vi "CRYStimulus Freq Max Limit.vi"(8 "Resolution":u16(ring) items=["R10 (1/3 Oct.)", "R20 (1/6 Oct.)", "R40 (1/12 Oct.)", "R80 (1/24 Oct.)", "User Defined, Log", "User Defined, Linear"], 9 "Decrement Flag":bool, 10 "Max Freq":dbl, 11 "Input Val":dbl) -> (2 "Decrement Val":dbl, 3 "Output Val":dbl)   [LabVIEW 2013]
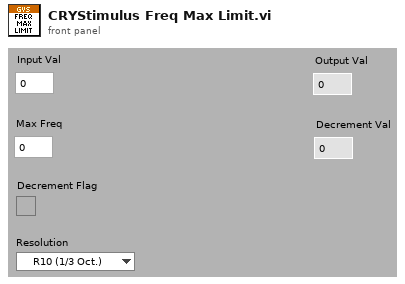
[diagram p1: front panel]
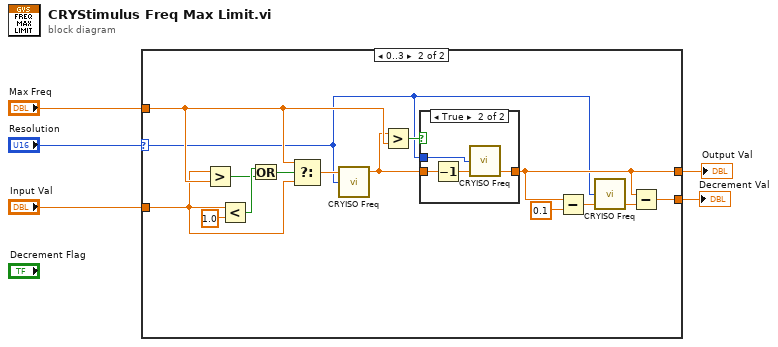
[diagram p0: block diagram]
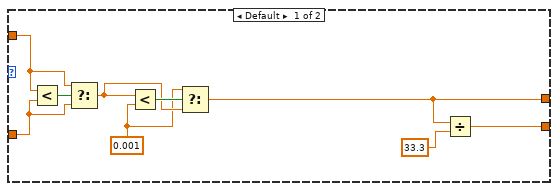
[diagram p2: hidden frame]
diagram:
  n1 = case shown="0..3" "Resolution" {
    selector: "Resolution" -> [_ w15]
    tunnel: [w6 w26] -> w5
    tunnel: [w8 w25] -> w4
    tunnel: "Max Freq" -> [w12 w23]
    tunnel: "Input Val" -> [w11 w22]
    frame Default {
      w9 = 0.001 ("y")
      n2 = Less?(x=w12, y=w11) -> (x < y?=w13:bool)
      n3 = Select(t=w12, s=w13, f=w11) -> (s? t:f=w10:dbl)
      n4 = Less?(x=w10, y=w9) -> (x < y?=w14:bool)
      n5 = Select(t=w9, s=w14, f=w10) -> (s? t:f=w8:dbl)
      n6 = Divide(x=w8, y=33.3) -> (x/y=w6:dbl)
    }
    frame 0..3 {
      n7 = Greater?(x=w22, y=w23) -> (0:w27:bool)
      n8 = Less?(x=w22, y=1.0) -> (x < y?=w28:bool)
      n9 = Or(x=w28, y=w27) -> (x .or. y?=w24:bool)
      n10 = Select(t=w23, s=w24, f=w22) -> (s? t:f=w21:dbl)
      n11 = call "CRYISO Freq.vi"("ISO series"=w15, "Higher Freq"=w21) -> ("Higher ISO Freq"=w19:dbl)  [unwired: 1 in, 2 out]
      n12 = Greater?(x=w19, y=w23) -> (0:w20:bool)
      n13 = case shown="True" w20 {
        tunnel: w19 -> [w30 w34]
        tunnel: [w30 w33] -> w25
        tunnel: w15 -> [_ w31]
        frame False {
        }
        frame True {
          n14 = Decrement(x=w34) -> (x-1=w32:dbl)
          n15 = call "CRYISO Freq.vi"("Lower Freq"=w32, "ISO series"=w31) -> ("Lower ISO Freq"=w33:dbl)  [unwired: 1 in, 2 out]
        }
      }
      n16 = Subtract(x=w25, y=0.1) -> (x-y=w17:dbl)
      n17 = call "CRYISO Freq.vi"("Lower Freq"=w17, "ISO series"=w15) -> ("Lower ISO Freq"=w18:dbl)  [unwired: 1 in, 2 out]
      n18 = Subtract(x=w25, y=w18) -> (x-y=w26:dbl)
    }
  }
  "Output Val" <- w4
  "Decrement Val" <- w5
